vi "LogIn.vi"(7 "Timeout":bool, 8 "error in (no error)":errorcluster, 9 "IsInitialLogin":bool, 10 "LastUserName":string, 11 "Sequence Context In":refnum<k7>) -> (0 "error out":errorcluster, 2 "logOut":bool, 3 "Report Text":string)   [LabVIEW 2019]
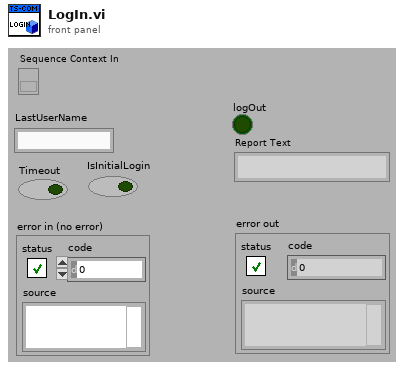
[diagram p1: front panel]
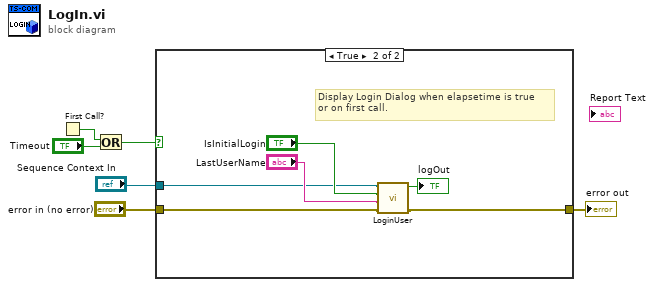
[diagram p0: block diagram]
diagram:
  n1 = First Call?() -> (First Call?: T/F=w2:bool)
  n2 = Or(x=w2, y="Timeout") -> (x .or. y?=w1:bool)
  n3 = case shown="True" w1 {
    tunnel: "error in (no error)" -> [w7 w13]
    tunnel: [w7 w12] -> w5
    tunnel: "Sequence Context In" -> [_ w9]
    frame False {
    }
    frame True {
      # "Display Login Dialog when elapsetime is true\nor on first call."
      n4 = call "LoginUser.vi"("error in (no error)"=w13, "LastUserName"="LastUserName", "IsInitialLogin"="IsInitialLogin", "Sequence Context In"=w9) -> ("error out"=w12:errorcluster, "logOut"=→"logOut":bool)  [unwired: 6 in]
    }
  }
  "error out" <- w5
